vi "Begin.vi"(8 "error in":errorcluster) -> (0 "error out":errorcluster)   [LabVIEW 2014]
doc: "Called before other user functions, this VI is expected to open initial I/O refnums, load in file data, and do all program initialization. Notice that the <B>error out</B> terminal is simply used for data flow. Wiring it to other structures or subVIs ensures that this VI runs first."
uses:
  <vilib>/Rock Robotics/WPI/DriverStation/WPI_DriverStationRobotMode2.ctl
  <vilib>/Rock Robotics/WPI/Joystick/WPI_JoystickDeviceEnum.ctl
  <vilib>/Rock Robotics/WPI/Solenoid/WPI_SolenoidChannel.ctl
  <vilib>/Rock Robotics/SystemInterfaces/DIO/FPGA_DIOChannel.ctl
  <vilib>/Rock Robotics/WPI/Encoder/WPI_EncoderType.ctl
  <vilib>/Rock Robotics/WPI/CAN/TalonSRX/WPI_CANTalonSRX_APIControlMode.ctl
  <vilib>/Rock Robotics/SystemInterfaces/Typedef/FPGA_TypedefDigitalModule.ctl
  <vilib>/Rock Robotics/SystemInterfaces/DIO/FPGA_DIOPWMChannel.ctl
  <vilib>/Rock Robotics/SystemInterfaces/Typedef/FPGA_TypedefAnalogModuleForGyro.ctl
  <vilib>/Rock Robotics/SystemInterfaces/AI/FPGA_AIGyroChannel.ctl
  Robot Global Data.vi
  <vilib>/Rock Robotics/WPI/Solenoid/WPI_SolenoidOpenDouble.vi
  <vilib>/Rock Robotics/WPI/Compressor/WPI_CompressorGetSetRefNum.vi
  <vilib>/Rock Robotics/WPI/MotorControl/WPI_MotorControlOpenCANTalonSRX.vi
  <vilib>/Rock Robotics/WPI/MotorControl/WPI_MotorControlOpen Talon.vi
  <vilib>/Rock Robotics/WPI/Counter/WPI_CounterDigitalInputToDigitalSource.vi
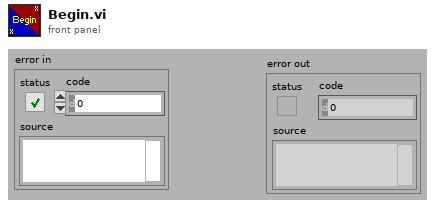
[diagram p1: front panel]
types:
  T1 = typedef "WPI_DriverStationRobotMode2.ctl" = enum16{"Autonomous Disabled", "Autonomous Enabled", "Teleop Disabled", "Teleop Enabled", "Disconnected", "Finish", "Test Disabled", "Test Enabled", "Emergency Stopped"}
  T2 = typedef "WPI_JoystickDeviceEnum.ctl" = enum16{"USB 0", "USB 1", "USB 2", "USB 3", "USB 4", "USB 5"}
  T3 = typedef "WPI_JoystickDevRef.ctl" = cluster{"Device":T2}
  T4 = typedef "FPGA_AIGyroChannel.ctl" = enum8{"AI 0", "AI 1", "Invalid"}
  T5 = typedef "FPGA_TypedefAnalogModuleForGyro.ctl" = enum16{"Controller 1"}
  T6 = typedef "WPI_GyroDevRef.ctl" = cluster{"DevStatus":errorcluster, "Analog Module":T7, "Analog Channel":T8, "Offset":dbl, "Gain (VoltsPerDegree/Second)":dbl}
  T7 = typedef "FPGA_TypedefAnalogModule.ctl" = enum16{"Controller 1"}
  T8 = typedef "FPGA_AIChannel.ctl" = enum8{"AI 0", "AI 1", "AI 2", "AI 3", "AI MXP 0", "AI MXP 1", "AI MXP 2", "AI MXP 3", "Invalid"}
  T9 = typedef "WPI_CompressorDevRef.ctl" = cluster{"DevStatus":errorcluster, "Pneumatics Control Module":u8}
  T10 = typedef "WPI_SolenoidChannel.ctl" = enum8{"Solenoid 0", "Solenoid 1", "Solenoid 2", "Solenoid 3", "Solenoid 4", "Solenoid 5", "Solenoid 6", "Solenoid 7", "Invalid"}
  T11 = typedef "WPI_SolenoidDevRef.ctl" = cluster{"DevStatus":errorcluster, "Pneumatics Control Module":u8, "Forward Solenoid Channel":T10, "Reverse Solenoid Channel":T10}
  T12 = typedef "FPGA_DIOPWMChannel.ctl" = enum8{"PWM 0", "PWM 1", "PWM 2", "PWM 3", "PWM 4", "PWM 5", "PWM 6", "PWM 7", "PWM 8", "PWM 9", "PWM MXP 0", "PWM MXP 1", "PWM MXP 2", "PWM MXP 3", "PWM MXP 4", "PWM MXP 5", "PWM MXP 6", "PWM MXP 7", "PWM MXP 8", "PWM MXP 9", "Invalid"}
  T13 = typedef "FPGA_TypedefDigitalModule.ctl" = enum16{"Controller 1"}
  T14 = typedef "WPI_CANTalonSRX_APIControlMode.ctl" = enum8{"Percent VBus", "Speed", "Position", "Slave", "Unchanged / Invalid"}
  T15 = typedef "WPI_MotorControlDeviceRef.ctl" = cluster{"DeviceStatus":errorcluster, "Type":T16, "PWM":cluster{"Controller":T13, "PWM Channel":T12, "DeadBand":T17}, "CAN":cluster{"Device Number":u8, "Control Mode":T18, "Semaphore":T19, "Max Vout":dbl, "TalonSRX Control Mode":T14}, "Invert":bool, "TransformRef":T20, "InvTransformRef":T20}
  T16 = typedef "WPI_MotorControlType.ctl" = enum16{"PWM", "CAN", "CANTalonSRX"}
  T17 = typedef "WPI_PWMDeadband.ctl" = cluster{"Name":string, "maxPositivePwm":i32, "minPositivePwm":i32, "centerPwm":i32, "maxNegativePwm":i32, "minNegativePwm":i32, "angularRange":u16}
  T18 = typedef "WPI_CANJaguar_ControlMode.ctl" = enum8{"Percent VBus", "Current", "Speed", "Position", "Voltage"}
  T19 = typedef "Semaphore RefNum" = refnum<k1>
  T20 = typedef "WPI_PWMTransform_ConPane.ctl" = refnum<vi>
  T21 = typedef "WPI_EncoderType.ctl" = enum16{"1x", "2x", "4x"}
  T22 = typedef "FPGA_DIOChannel.ctl" = enum8{"DIO 0", "DIO 1", "DIO 2", "DIO 3", "DIO 4", "DIO 5", "DIO 6", "DIO 7", "DIO 8", "DIO 9", "DIO MXP 0", "DIO MXP 1", "DIO MXP 2", "DIO MXP 3", "DIO MXP 4", "DIO MXP 5", "DIO MXP 6", "DIO MXP 7", "DIO MXP 8", "DIO MXP 9", "DIO MXP 10", "DIO MXP 11", "DIO MXP 12", "DIO MXP 13", "DIO MXP 14", "DIO MXP 15", "Invalid"}
  T23 = typedef "WPI_DigitalInputDevRef.ctl" = cluster{"DevStatus":errorcluster, "DIO Channel":T22, "Controller":T13}
  T24 = typedef "FPGA_CounterEncoderSourceConvertionLVSourceType.ctl" = cluster{"DevStatus":errorcluster, "AnalogTriggerMode?":bool, "DigitalMode":cluster{"Controller":T13, "DIO Channel":T25}, "AnalogTriggerMode":cluster{"AnalogTriggerIndex":T26, "OutputType":T27}}
  T25 = typedef "FPGA_DIODigitalSourceChannel.ctl" = enum8{"DIO 0", "DIO 1", "DIO 2", "DIO 3", "DIO 4", "DIO 5", "DIO 6", "DIO 7", "DIO 8", "DIO 9", "DIO MXP 0", "DIO MXP 1", "DIO MXP 2", "DIO MXP 3", "DIO MXP 4", "DIO MXP 5", "DIO MXP 6", "DIO MXP 7", "DIO MXP 8", "DIO MXP 9", "DIO MXP 10", "DIO MXP 11", "DIO MXP 12", "DIO MXP 13", "DIO MXP 14", "DIO MXP 15", "Disabled"}
  T26 = typedef "FPGA_AnalogTriggerIndex.ctl" = enum8{"Trig 0", "Trig 1", "Trig 2", "Trig 3", "Trig 4", "Trig 5", "Trig 6", "Trig 7", "Invalid"}
  T27 = typedef "FPGA_AnalogTriggerOutType.ctl" = enum16{"InWindow", "TriggerState", "Rising", "Falling"}
  T28 = typedef "WPI_EncoderDevRef.ctl" = cluster{"DevStatus":errorcluster, "EncoderIndex":T29, "CounterIndex":T30, "DistancePerCount":dbl, "Decoding Type":T21}
  T29 = typedef "FPGA_EncoderIdx.ctl" = enum8{"Enc 0", "Enc 1", "Enc 2", "Enc 3", "Enc 4", "Enc 5", "Enc 6", "Enc 7", "Invalid"}
  T30 = typedef "FPGA_CounterCtrSystemIndex.ctl" = enum8{"Ctr 0", "Ctr 1", "Ctr 2", "Ctr 3", "Ctr 4", "Ctr 5", "Ctr 6", "Ctr 7", "Invalid"}
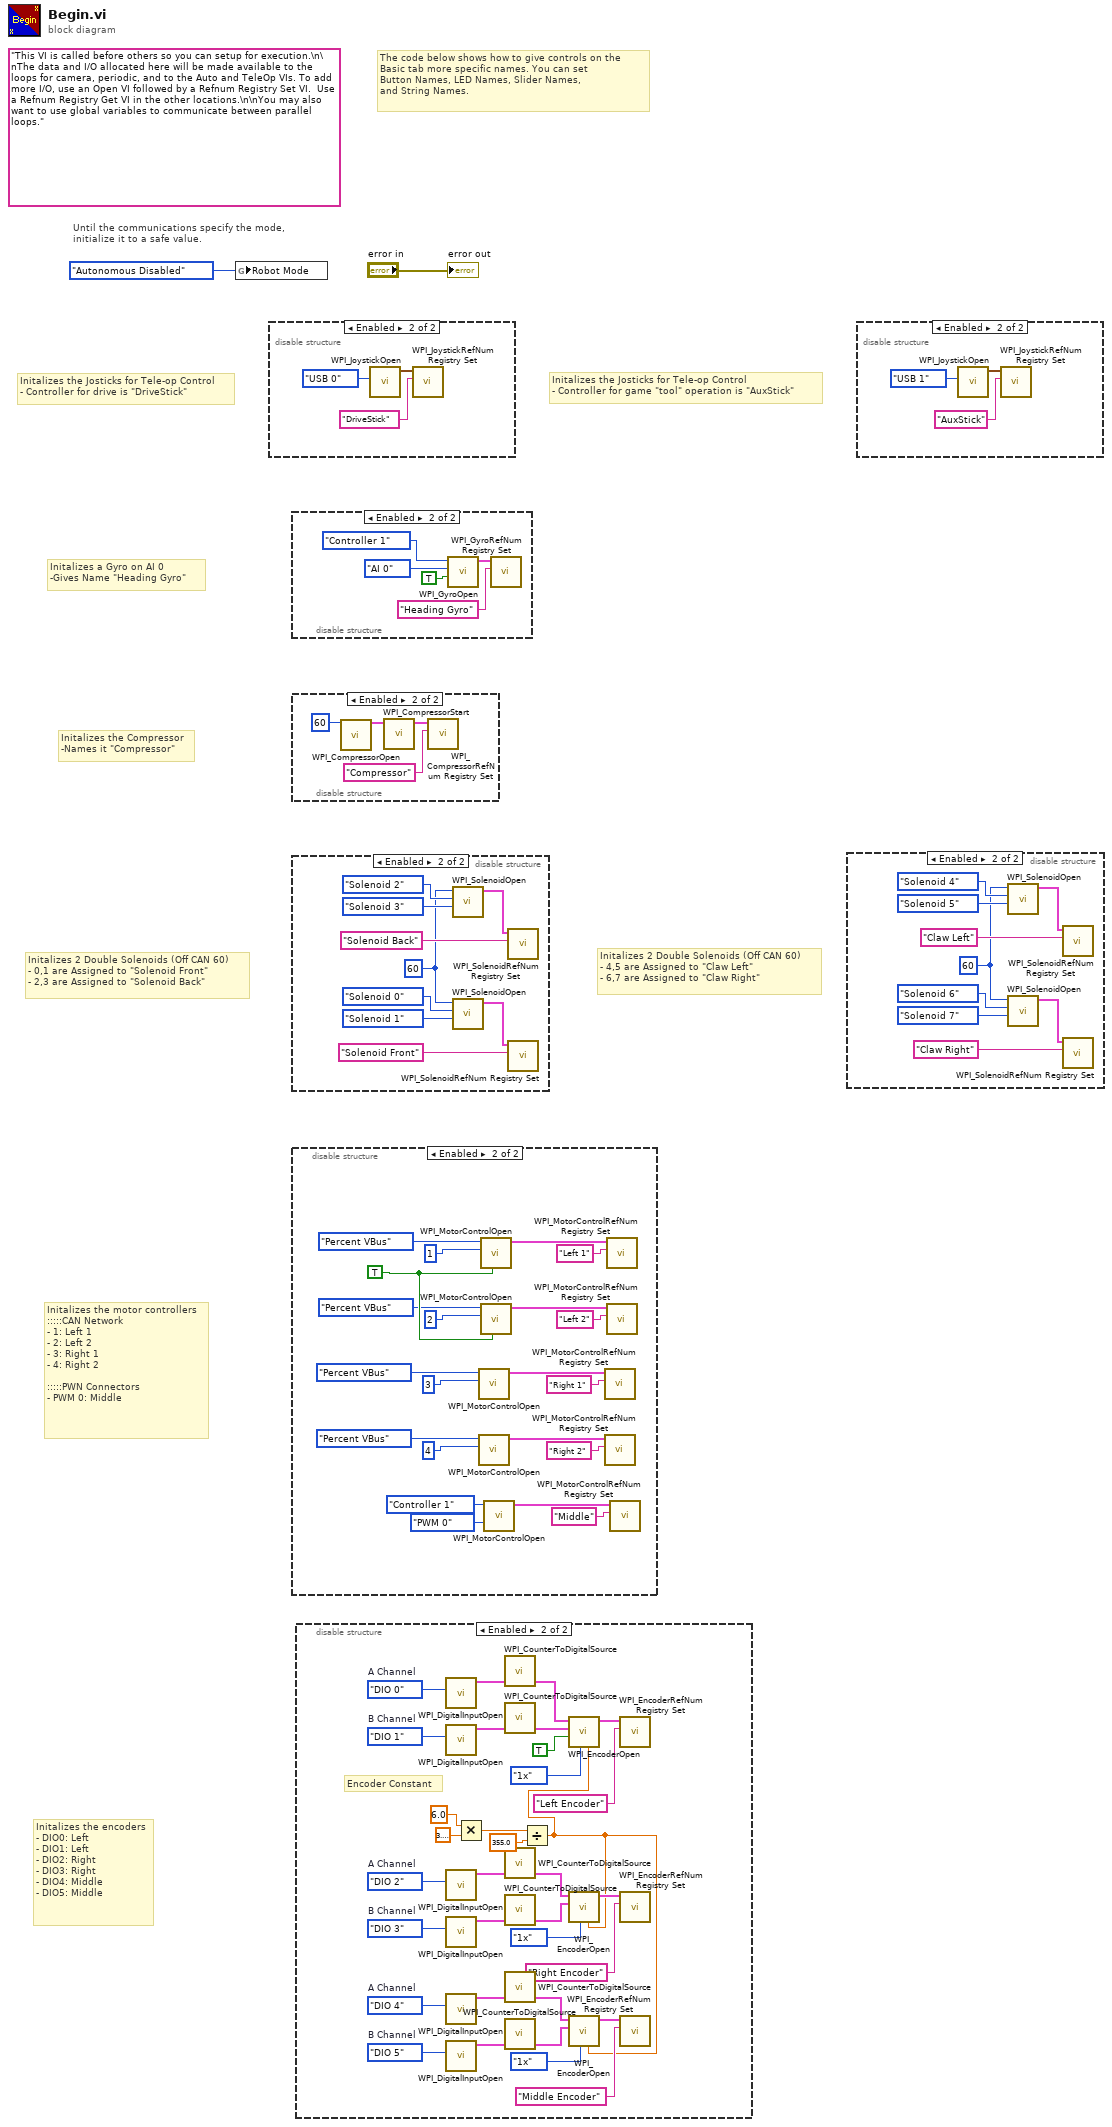
[diagram p0: block diagram]
diagram:
  (unwired) "This VI is called before others so you can setup for execution.\n\nThe data and I/O allocated here will be made available to the loops for camera, periodic, and to the Auto and TeleOp VIs. To add more I/O, use an Open VI followed by a Refnum Registry Set VI.  Use a Refnum Registry Get VI in the other locations.\n\nYou may also want to use global variables to communicate between parallel loops."
  # "Initalizes the Josticks for Tele-op Control\n- Controller for game \"tool\" operation is \"AuxStick\""
  # "Initalizes 2 Double Solenoids (Off CAN 60)\n- 4,5 are Assigned to \"Claw Left\"\n- 6,7 are Assigned to \"Claw Right\""
  # "Initalizes the encoders\n- DIO0: Left\n- DIO1: Left\n- DIO2: Right\n- DIO3: Right\n- DIO4: Middle\n- DIO5: Middle"
  # "Initalizes the motor controllers\n:::::CAN Network\n- 1: Left 1\n- 2: Left 2\n- 3: Right 1\n- 4: Right 2\n\n:::::PWN Connectors\n- PWM 0: Middle"
  # "Initalizes the Josticks for Tele-op Control\n- Controller for drive is \"DriveStick\""
  # "Initalizes the Compressor\n-Names it \"Compressor\""
  # "Initalizes 2 Double Solenoids (Off CAN 60)\n- 0,1 are Assigned to \"Solenoid Front\"\n- 2,3 are Assigned to \"Solenoid Back\""
  # "Initalizes a Gyro on AI 0\n-Gives Name \"Heading Gyro\""
  # "The code below shows how to give controls on the\nBasic tab more specific names. You can set\nButton Names, LED Names, Slider Names,\nand String Names."
  # "Until the communications specify the mode,\ninitialize it to a safe value."
  n1 = global write "Robot Global Data.vi" "Robot Mode"(WPI_DriverStationRobotMode2."Autonomous Disabled" ("Robot Mode")) -> ()
  n2 = disable-structure shown="Enabled" {
    frame Disabled {
    }
    frame Enabled {
      n3 = call <vilib>:"WPI_JoystickOpen.vi"("JoystickDevice"=WPI_JoystickDeviceEnum."USB 0") -> ("JoystickDevRef"=w4:T3)  [unwired: 10 in]
      n4 = call <vilib>:"WPI_JoystickRefNum Registry Set.vi"("refnum name"="DriveStick", "JoystickDevRef"=w4) -> ()  [unwired: 8 in, 2 out]
    }
  }
  n5 = disable-structure shown="Enabled" {
    frame Disabled {
    }
    frame Enabled {
      n6 = call <vilib>:"WPI_GyroOpen.vi"("Calibrate On Open"=TRUE, "Analog Channel"=FPGA_AIGyroChannel."AI 0", "Controller"=FPGA_TypedefAnalogModuleForGyro."Controller 1") -> ("GyroDevRef"=w9:T6)  [unwired: 6 in, 2 out]
      n7 = call <vilib>:"WPI_GyroRefNum Registry Set.vi"("refnum name"="Heading Gyro", "GyroDevRef"=w9) -> ()  [unwired: 8 in, 2 out]
    }
  }
  n8 = disable-structure shown="Enabled" {
    frame Disabled {
    }
    frame Enabled {
      n9 = call <vilib>:"WPI_CompressorOpen.vi"("Pneumatics Control Module (0)"=u8 60) -> ("CompressorDevRef"=w13:T9)  [unwired: 13 in, 1 out]
      n10 = call <vilib>:"WPI_CompressorStart.vi"("CompressorDevRef"=w13) -> ("CompressorDevRef"=w14:T9)  [unwired: 9 in, 1 out]
      n11 = call <vilib>:"WPI_CompressorRefNum Registry Set.vi"("refnum name"="Compressor", "CompressorDevRef"=w14) -> ()  [unwired: 8 in, 2 out]
    }
  }
  n12 = disable-structure shown="Enabled" {
    frame Disabled {
    }
    frame Enabled {
      w15 = u8 60 ("Pneumatics Control Module (0)")
      n13 = call-poly <vilib>:"WPI_SolenoidOpen.vi"("Reverse Solenoid Channel"=WPI_SolenoidChannel."Solenoid 3", "Forward Solenoid Channel"=WPI_SolenoidChannel."Solenoid 2", "Pneumatics Control Module (0)"=w15) -> ("SolenoidDevRef"=w21:T11)  [unwired: 7 in, 1 out]
      n14 = call-poly <vilib>:"WPI_SolenoidOpen.vi"("Reverse Solenoid Channel"=WPI_SolenoidChannel."Solenoid 1", "Forward Solenoid Channel"=WPI_SolenoidChannel."Solenoid 0", "Pneumatics Control Module (0)"=w15) -> ("SolenoidDevRef"=w20:T11)  [unwired: 7 in, 1 out]
      n15 = call <vilib>:"WPI_SolenoidRefNum Registry Set.vi"("refnum name"="Solenoid Back", "SolenoidDevRef"=w21) -> ()  [unwired: 8 in, 2 out]
      n16 = call <vilib>:"WPI_SolenoidRefNum Registry Set.vi"("refnum name"="Solenoid Front", "SolenoidDevRef"=w20) -> ()  [unwired: 8 in, 2 out]
    }
  }
  n17 = disable-structure shown="Enabled" {
    frame Disabled {
    }
    frame Enabled {
      w44 = TRUE ("Invert")
      n18 = call-poly <vilib>:"WPI_MotorControlOpen.vi"("Device Number"=u8 3, "Control Mode"=WPI_CANTalonSRX_APIControlMode."Percent VBus") -> ("MotorControlDeviceRef"=w36:T15)  [unwired: 8 in, 1 out]
      n19 = call-poly <vilib>:"WPI_MotorControlOpen.vi"("Device Number"=u8 4, "Control Mode"=WPI_CANTalonSRX_APIControlMode."Percent VBus") -> ("MotorControlDeviceRef"=w37:T15)  [unwired: 8 in, 1 out]
      n20 = call-poly <vilib>:"WPI_MotorControlOpen.vi"("Invert"=w44, "Device Number"=u8 1, "Control Mode"=WPI_CANTalonSRX_APIControlMode."Percent VBus") -> ("MotorControlDeviceRef"=w28:T15)  [unwired: 7 in, 1 out]
      n21 = call-poly <vilib>:"WPI_MotorControlOpen.vi"("Invert"=w44, "Device Number"=u8 2, "Control Mode"=WPI_CANTalonSRX_APIControlMode."Percent VBus") -> ("MotorControlDeviceRef"=w29:T15)  [unwired: 7 in, 1 out]
      n22 = call-poly <vilib>:"WPI_MotorControlOpen.vi"("PWM Channel"=FPGA_DIOPWMChannel."PWM 0", "Controller"=FPGA_TypedefDigitalModule."Controller 1") -> ("MotorControlDeviceRef"=w40:T15)  [unwired: 8 in, 1 out]
      n23 = call <vilib>:"WPI_MotorControlRefNum Registry Set.vi"("refnum name"="Right 1", "MotorControlDevRef"=w36) -> ()  [unwired: 8 in, 2 out]
      n24 = call <vilib>:"WPI_MotorControlRefNum Registry Set.vi"("refnum name"="Right 2", "MotorControlDevRef"=w37) -> ()  [unwired: 8 in, 2 out]
      n25 = call <vilib>:"WPI_MotorControlRefNum Registry Set.vi"("refnum name"="Left 1", "MotorControlDevRef"=w28) -> ()  [unwired: 8 in, 2 out]
      n26 = call <vilib>:"WPI_MotorControlRefNum Registry Set.vi"("refnum name"="Left 2", "MotorControlDevRef"=w29) -> ()  [unwired: 8 in, 2 out]
      n27 = call <vilib>:"WPI_MotorControlRefNum Registry Set.vi"("refnum name"="Middle", "MotorControlDevRef"=w40) -> ()  [unwired: 8 in, 2 out]
    }
  }
  n28 = disable-structure shown="Enabled" {
    frame Disabled {
    }
    frame Enabled {
      w61 = FPGA_DIOChannel."DIO 5"  # B Channel
      w60 = FPGA_DIOChannel."DIO 4"  # A Channel
      w69 = FPGA_DIOChannel."DIO 3"  # B Channel
      w68 = FPGA_DIOChannel."DIO 2"  # A Channel
      w77 = FPGA_DIOChannel."DIO 1"  # B Channel
      w76 = FPGA_DIOChannel."DIO 0"  # A Channel
      # "Encoder Constant"
      n29 = call <vilib>:"WPI_DigitalInputOpen.vi"("DIO Channel"=w76) -> ("DigitalInputDevRef"=w73:T23)  [unwired: 2 in, 8 out]
      n30 = call <vilib>:"WPI_DigitalInputOpen.vi"("DIO Channel"=w77) -> ("DigitalInputDevRef"=w74:T23)  [unwired: 2 in, 8 out]
      n31 = call <vilib>:"WPI_DigitalInputOpen.vi"("DIO Channel"=w68) -> ("DigitalInputDevRef"=w65:T23)  [unwired: 2 in, 8 out]
      n32 = call <vilib>:"WPI_DigitalInputOpen.vi"("DIO Channel"=w69) -> ("DigitalInputDevRef"=w66:T23)  [unwired: 2 in, 8 out]
      n33 = call <vilib>:"WPI_DigitalInputOpen.vi"("DIO Channel"=w60) -> ("DigitalInputDevRef"=w57:T23)  [unwired: 2 in, 8 out]
      n34 = call <vilib>:"WPI_DigitalInputOpen.vi"("DIO Channel"=w61) -> ("DigitalInputDevRef"=w58:T23)  [unwired: 2 in, 8 out]
      n35 = Multiply(x=6.0, y=3.141592653589793) -> (x*y=w50:dbl)
      n36 = call-poly <vilib>:"WPI_CounterToDigitalSource.vi"("DigitalInputDevRef"=w73) -> ("Digital Source"=w72:T24)  [unwired: 6 out]
      n37 = call-poly <vilib>:"WPI_CounterToDigitalSource.vi"("DigitalInputDevRef"=w74) -> ("Digital Source"=w75:T24)  [unwired: 6 out]
      n38 = call-poly <vilib>:"WPI_CounterToDigitalSource.vi"("DigitalInputDevRef"=w65) -> ("Digital Source"=w64:T24)  [unwired: 6 out]
      n39 = call-poly <vilib>:"WPI_CounterToDigitalSource.vi"("DigitalInputDevRef"=w66) -> ("Digital Source"=w67:T24)  [unwired: 6 out]
      n40 = call-poly <vilib>:"WPI_CounterToDigitalSource.vi"("DigitalInputDevRef"=w57) -> ("Digital Source"=w56:T24)  [unwired: 6 out]
      n41 = call-poly <vilib>:"WPI_CounterToDigitalSource.vi"("DigitalInputDevRef"=w58) -> ("Digital Source"=w59:T24)  [unwired: 6 out]
      n42 = Divide(x=w50, y=355.0) -> (x/y=w48:dbl)
      n43 = call <vilib>:"WPI_EncoderOpen.vi"("DistancePerCount"=w48, "Decoding Type"=WPI_EncoderType."1x", "Invert Direction (False)"=TRUE, "BSource"=w75, "ASource"=w72) -> ("EncoderDevRef"=w71:T28)  [unwired: 3 in, 3 out]
      n44 = call <vilib>:"WPI_EncoderOpen.vi"("DistancePerCount"=w48, "Decoding Type"=WPI_EncoderType."1x", "BSource"=w67, "ASource"=w64) -> ("EncoderDevRef"=w63:T28)  [unwired: 4 in, 3 out]
      n45 = call <vilib>:"WPI_EncoderOpen.vi"("DistancePerCount"=w48, "Decoding Type"=WPI_EncoderType."1x", "BSource"=w59, "ASource"=w56) -> ("EncoderDevRef"=w55:T28)  [unwired: 4 in, 3 out]
      n46 = call <vilib>:"WPI_EncoderRefNum Registry Set.vi"("refnum name"="Left Encoder", "EncoderDevRef"=w71) -> ()  [unwired: 8 in, 2 out]
      n47 = call <vilib>:"WPI_EncoderRefNum Registry Set.vi"("refnum name"="Right Encoder", "EncoderDevRef"=w63) -> ()  [unwired: 8 in, 2 out]
      n48 = call <vilib>:"WPI_EncoderRefNum Registry Set.vi"("refnum name"="Middle Encoder", "EncoderDevRef"=w55) -> ()  [unwired: 8 in, 2 out]
    }
  }
  n49 = disable-structure shown="Enabled" {
    frame Disabled {
    }
    frame Enabled {
      w78 = u8 60 ("Pneumatics Control Module (0)")
      n50 = call-poly <vilib>:"WPI_SolenoidOpen.vi"("Reverse Solenoid Channel"=WPI_SolenoidChannel."Solenoid 5", "Forward Solenoid Channel"=WPI_SolenoidChannel."Solenoid 4", "Pneumatics Control Module (0)"=w78) -> ("SolenoidDevRef"=w84:T11)  [unwired: 7 in, 1 out]
      n51 = call-poly <vilib>:"WPI_SolenoidOpen.vi"("Reverse Solenoid Channel"=WPI_SolenoidChannel."Solenoid 7", "Forward Solenoid Channel"=WPI_SolenoidChannel."Solenoid 6", "Pneumatics Control Module (0)"=w78) -> ("SolenoidDevRef"=w83:T11)  [unwired: 7 in, 1 out]
      n52 = call <vilib>:"WPI_SolenoidRefNum Registry Set.vi"("refnum name"="Claw Left", "SolenoidDevRef"=w84) -> ()  [unwired: 8 in, 2 out]
      n53 = call <vilib>:"WPI_SolenoidRefNum Registry Set.vi"("refnum name"="Claw Right", "SolenoidDevRef"=w83) -> ()  [unwired: 8 in, 2 out]
    }
  }
  n54 = disable-structure shown="Enabled" {
    frame Disabled {
    }
    frame Enabled {
      n55 = call <vilib>:"WPI_JoystickOpen.vi"("JoystickDevice"=WPI_JoystickDeviceEnum."USB 1") -> ("JoystickDevRef"=w88:T3)  [unwired: 10 in]
      n56 = call <vilib>:"WPI_JoystickRefNum Registry Set.vi"("refnum name"="AuxStick", "JoystickDevRef"=w88) -> ()  [unwired: 8 in, 2 out]
    }
  }
  "error out" <- "error in"
